vi "Stop Acquisition.vi"(8 "error in (no error)":errorcluster, 11 "Hardware Resources in":T1) -> (0 "error out":errorcluster)   [LabVIEW 2013, in "Logging Acquisition.lvlib"]
doc: "Stops the acquisition."
uses:
  Logging Acquisition.lvlib
  Hardware Configuration.ctl
  Signal Type.ctl
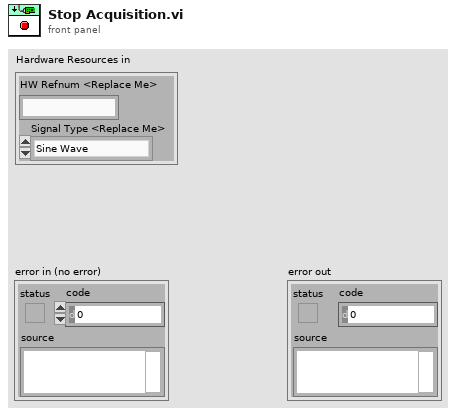
[diagram p1: front panel]
types:
  T1 = typedef "Logging Acquisition.lvlib/Hardware Configuration.ctl" = cluster{"HW Refnum <Replace Me>":string, "Signal Type <Replace Me>":T2}
  T2 = typedef "Logging Acquisition.lvlib/Signal Type.ctl" = enum16{"Sine Wave", "Square with Noise"}
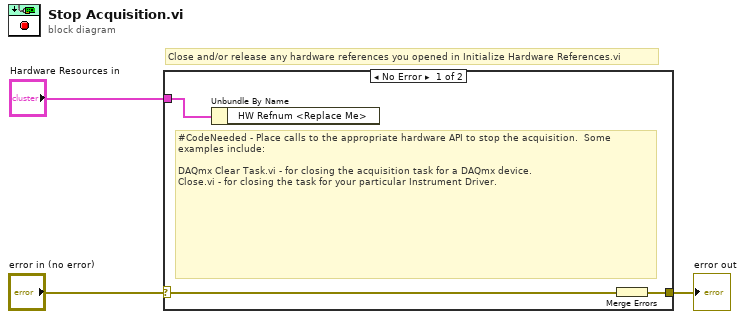
[diagram p0: block diagram]
diagram:
  # "Close and/or release any hardware references you opened in Initialize Hardware References.vi"
  n1 = case shown="No Error" "error in (no error)" {
    selector: "error in (no error)" -> [w5 w7]
    tunnel: [w6 w7] -> w2
    tunnel: "Hardware Resources in" -> [w4 _]
    frame No Error {
      # "#CodeNeeded - Place calls to the appropriate hardware API to stop the acquisition.  Some examples include:\n\nDAQmx Clear Task.vi - for closing the acquisition task for a DAQmx device.\nClose.vi - for closing the task for your particular Instrument Driver."
      n2 = Unbundle By Name(w4) -> ()  [unwired: 1 out]
      n3 = Merge Errors(w5) -> (w6:errorcluster)
    }
    frame Error {
    }
  }
  "error out" <- w2
